vi "FlatToRichcif_manager_UnregisterPluginRequest.vi"(5 "OutputClusterType":T1, 11 "InputCluster":T2) -> (3 "OutputCluster":T1)   [LabVIEW 2021, in "CIF_Manager_server.lvlib"]
uses:
  CIF_Manager_server.lvlib
  cif_manager_UnregisterPluginRequest_Flat.ctl
  cif_manager_UnregisterPluginRequest.ctl
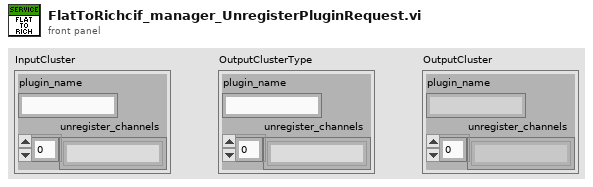
[diagram p1: front panel]
types:
  T1 = typedef "CIF_Manager_server.lvlib/cif_manager_UnregisterPluginRequest.ctl" = cluster{"plugin_name":string, "unregister_channels":string[]}
  T2 = typedef "CIF_Manager_server.lvlib/cif_manager_UnregisterPluginRequest_Flat.ctl" = cluster{"plugin_name":string, "unregister_channels":string[]}
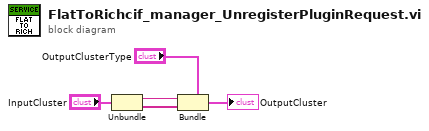
[diagram p0: block diagram]
diagram:
  n1 = Unbundle "Unbundle"("InputCluster") -> ("plugin_name"=w2:string, "unregister_channels"=w1:string[])
  n2 = Bundle "Bundle"(cluster="OutputClusterType", "plugin_name"=w2, "unregister_channels"=w1) -> (→"OutputCluster":T1)
